vi "GetButtonHelpText.vi"(0 "reference in":refnum<class "DqmhModuleDiagramGraph.lvclass">, 2 "ButtonString":string, 5 "error in (no error)":errorcluster) -> (14 "reference out":refnum<class "DqmhModuleDiagramGraph.lvclass">, 16 "HelpOut":T1, 19 "error out":errorcluster)   [LabVIEW 2020, in "DqmhModuleDiagramGraph.lvclass"]
uses:
  <resource>/Framework/Providers/Open_GDS/UML/DqmhModuleDiagramGraph_class/DqmhModuleDiagramGraph.lvclass
  <resource>/Framework/Providers/Open_GDS/UML/ContextHelp/ContextHelp_ShowType.ctl
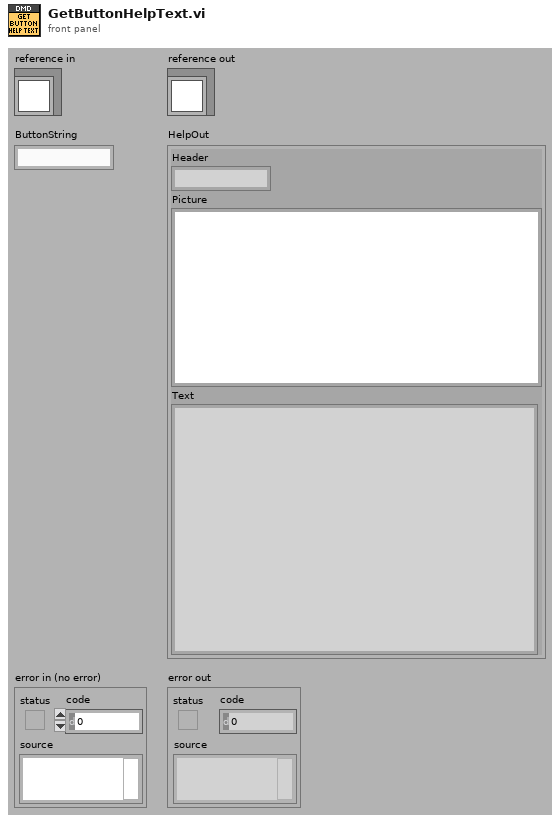
[diagram p1: front panel]
types:
  T1 = typedef "ContextHelp_ShowType.ctl" = cluster{"Header":string, "Picture":picture, "Text":string}
  T2 = typedef "Graph.lvclass/ToolbarButtonType.ctl" = cluster{"Text":string, "Type":T3}
  T3 = typedef "UMLEditor tooltype.ctl" = enum16{"None", "Node", "Edge"}
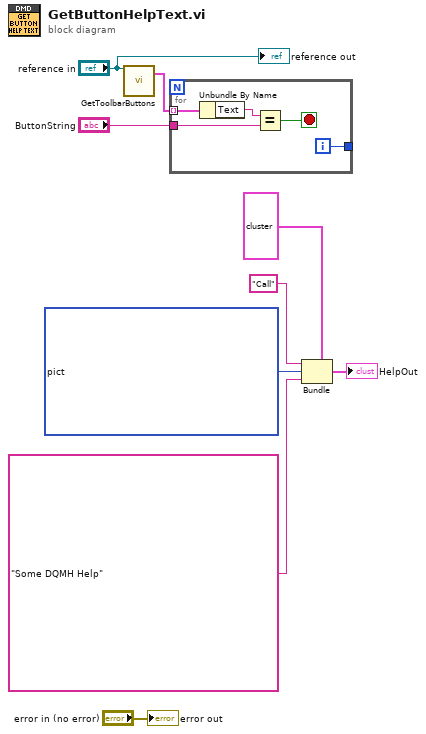
[diagram p0: block diagram]
diagram:
  n1 = call-dynamic "GetToolbarButtons.vi"("reference in"="reference in") -> ("ToolbarButtons"=w7:T2[])  [unwired: 14 in, 4 out]
  n2 = for {
    tunnel: w7 -> [w14] mode=indexing
    tunnel: "ButtonString" -> [w12]
    tunnel: [w10] -> _
    i -> [w10]
    stop <- w11 stop-if-true
    n3 = Unbundle By Name(w14) -> ("Text"=w13:string)
    n4 = Equal?(x=w13, y=w12) -> (x = y?=w11:bool)
  }
  n5 = Bundle(cluster=cluster{string, "empty picture":picture, string} {"", "empty picture"=bytes[0], ""}, "Call", "empty picture"=picture bytes[165420] ("Picture"), "Some DQMH Help") -> (→"HelpOut":cluster{string, "empty picture":picture, string})
  "error out" <- "error in (no error)"
  "reference out" <- "reference in"
